vi "DataRecording_Header.vi"(0 "User":string, 1 "StartDate":string, 2 "StartTime":string, 3 "Bursting Mode":string, 4 "Flow Rate Level":i32, 5 "Experiment Infos":string, 6 "Test Name":string, 7 "StartPressure":string) -> (14 "Header":string)   [LabVIEW 2020]
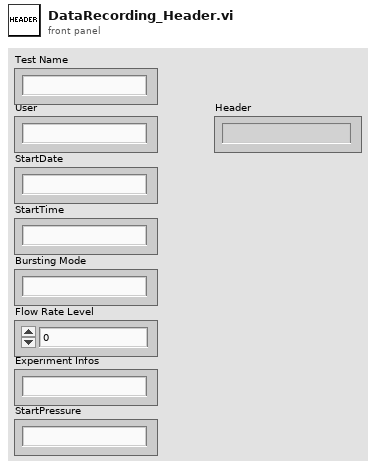
[diagram p1: front panel]
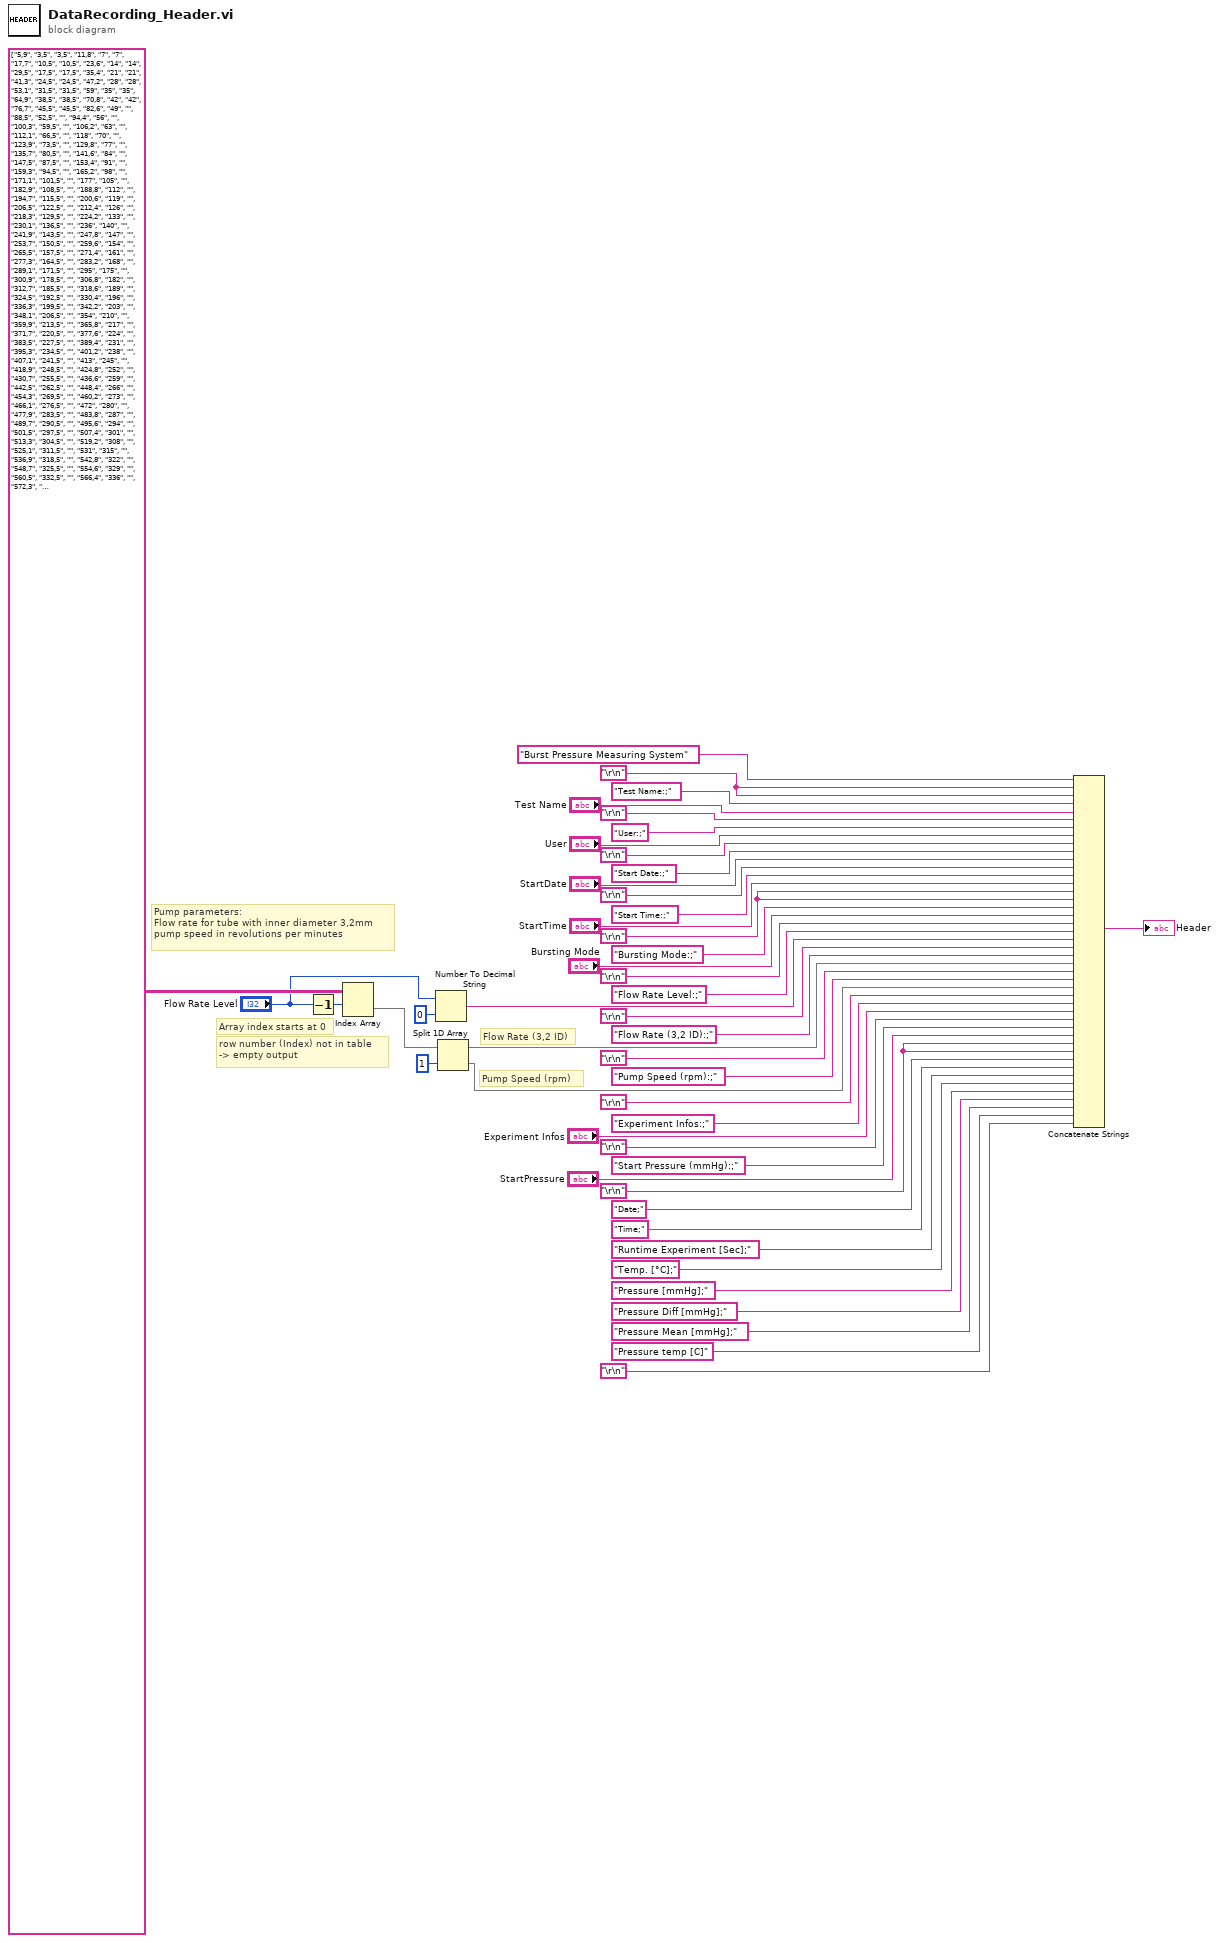
[diagram p0: block diagram]
diagram:
  w22 = "\r\n"
  w31 = "\r\n"
  w34 = "\r\n"
  # "row number (Index) not in table\n-> empty output"
  # "Pump Speed (rpm)"
  # "Flow Rate (3,2 ID)"
  # "Pump parameters:\nFlow rate for tube with inner diameter 3,2mm\npump speed in revolutions per minutes"
  # "Array index starts at 0"
  n1 = Decrement(x="Flow Rate Level") -> (x-1=w12:i32)
  n2 = Index Array(array=string[][] [["5,9", "3,5", "3,5"], ["11,8", "7", "7"], ["17,7", "10,5", "10,5"], ["23,6", "14", "14"], ["29,5", "17,5", "17,5"], ["35,4", "21", "21"], ["41,3", "24,5", "24,5"], ["47,2", "28", "28"], ["53,1", "31,5", "31,5"], ["59", "35", "35"], ["64,9", "38,5", "38,5"], ["70,8", "42", "42"], ["76,7", "45,5", "45,5"], ["82,6", "49", ""], ["88,5", "52,5", ""], ["94,4", "56", ""], ["100,3", "59,5", ""], ["106,2", "63", ""], ["112,1", "66,5", ""], ["118", "70", ""], ["123,9", "73,5", ""], ["129,8", "77", ""], ["135,7", "80,5", ""], ["141,6", "84", ""], ["147,5", "87,5", ""], ["153,4", "91", ""], ["159,3", "94,5", ""], ["165,2", "98", ""], ["171,1", "101,5", ""], ["177", "105", ""], ["182,9", "108,5", ""], ["188,8", "112", ""], ["194,7", "115,5", ""], ["200,6", "119", ""], ["206,5", "122,5", ""], ["212,4", "126", ""], ["218,3", "129,5", ""], ["224,2", "133", ""], ["230,1", "136,5", ""], ["236", "140", ""], ["241,9", "143,5", ""], ["247,8", "147", ""], ["253,7", "150,5", ""], ["259,6", "154", ""], ["265,5", "157,5", ""], ["271,4", "161", ""], ["277,3", "164,5", ""], ["283,2", "168", ""], ["289,1", "171,5", ""], ["295", "175", ""], ["300,9", "178,5", ""], ["306,8", "182", ""], ["312,7", "185,5", ""], ["318,6", "189", ""], ["324,5", "192,5", ""], ["330,4", "196", ""], ["336,3", "199,5", ""], ["342,2", "203", ""], ["348,1", "206,5", ""], ["354", "210", ""], ["359,9", "213,5", ""], ["365,8", "217", ""], ["371,7", "220,5", ""], ["377,6", "224", ""], ["383,5", "227,5", ""], ["389,4", "231", ""], ["395,3", "234,5", ""], ["401,2", "238", ""], ["407,1", "241,5", ""], ["413", "245", ""], ["418,9", "248,5", ""], ["424,8", "252", ""], ["430,7", "255,5", ""], ["436,6", "259", ""], ["442,5", "262,5", ""], ["448,4", "266", ""], ["454,3", "269,5", ""], ["460,2", "273", ""], ["466,1", "276,5", ""], ["472", "280", ""], ["477,9", "283,5", ""], ["483,8", "287", ""], ["489,7", "290,5", ""], ["495,6", "294", ""], ["501,5", "297,5", ""], ["507,4", "301", ""], ["513,3", "304,5", ""], ["519,2", "308", ""], ["525,1", "311,5", ""], ["531", "315", ""], ["536,9", "318,5", ""], ["542,8", "322", ""], ["548,7", "325,5", ""], ["554,6", "329", ""], ["560,5", "332,5", ""], ["566,4", "336", ""], ["572,3", "339,5", ""], ["578,2", "343", ""], ["584,1", "346,5", ""]], index (row)=w12) -> (element=w7:string[])  [unwired: 1 in]
  n3 = Number To Decimal String(number="Flow Rate Level", width (-)=i16 0) -> (decimal integer string=w10:string)
  n4 = Split 1D Array(array=w7, index=1) -> (first subarray=w5:string[], second subarray=w4:string[])
  n5 = Concatenate Strings("Burst Pressure Measuring System" ("string"), w34, w34, "Test Name:;" ("string"), "Test Name", "\r\n", "User:;" ("string"), "User", "\r\n", "Start Date:;" ("string"), "StartDate", "\r\n", "Start Time:;" ("string"), "StartTime", w31, w31, "Bursting Mode:;" ("string"), "Bursting Mode", "\r\n", "Flow Rate Level:;" ("string"), w10, "\r\n", "Flow Rate (3,2 ID):;" ("string"), w5, "\r\n", "Pump Speed (rpm):;" ("string"), w4, "\r\n", "Experiment Infos:;" ("string"), "Experiment Infos", "\r\n", "Start Pressure (mmHg):;" ("string"), "StartPressure", w22, w22, "Date;" ("string"), "Time;" ("string"), "Runtime Experiment [Sec];" ("string"), "Temp. [°C];" ("string"), "Pressure [mmHg];" ("string"), "Pressure Diff [mmHg];" ("string"), "Pressure Mean [mmHg];" ("string"), "Pressure temp [C]" ("string"), "\r\n") -> (→"Header":string)
